vi "PathHeadingCalculator.vi"(1 "yi1":dbl format="%#_13g", 2 "xi1":dbl format="%#_13g", 3 "yi":dbl format="%#_13g", 4 "xi":dbl format="%#_13g") -> (0 "PathHeading":dbl)   [LabVIEW 2024]
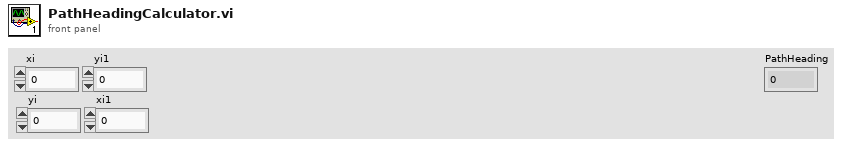
[diagram p1: front panel]
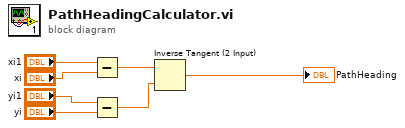
[diagram p0: block diagram]
diagram:
  n1 = Subtract(x="xi1", y="xi") -> (x-y=w3:dbl)
  n2 = Subtract(x="yi1", y="yi") -> (x-y=w2:dbl)
  n3 = Inverse Tangent (2 Input)(1:w2, 2:w3) -> (0:→"PathHeading":dbl)
